vi "Check All.vi"(8 "error in (no error)":errorcluster, 11 "Lamp Container in":refnum<class "Lamp Container.lvclass">) -> (0 "error out":errorcluster, 3 "Lamp Container out":refnum<class "Lamp Container.lvclass">)   [LabVIEW 2016, in "Lamp Container.lvclass"]
uses:
  Lamp Container.lvclass
  Lamp Container.lvclass/Lamp Container.ctl
  ThAr/ThAr.lvclass
  LED/LED.lvclass
  Quartz/Quartz.lvclass
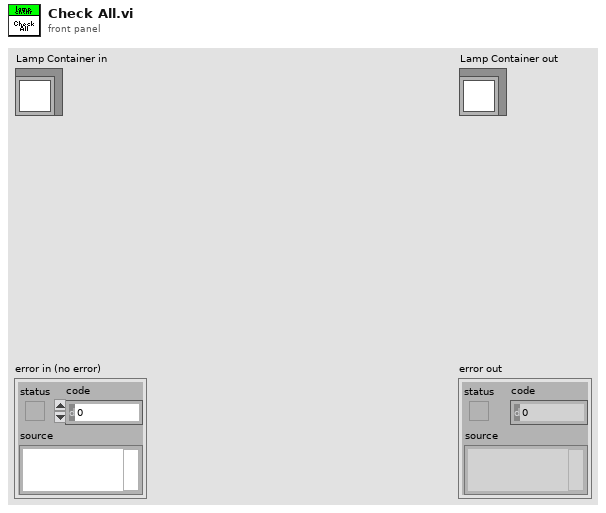
[diagram p1: front panel]
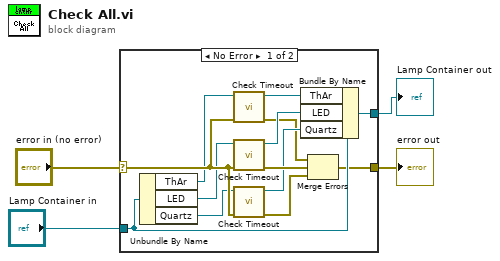
[diagram p0: block diagram]
diagram:
  n1 = case shown="No Error" "error in (no error)" {
    selector: "error in (no error)" -> [w14 w19]
    tunnel: [w15 w19] -> w3
    tunnel: [w16 w18] -> w1
    tunnel: "Lamp Container in" -> [w17 w18]
    frame No Error {
      n2 = Unbundle By Name(w17) -> ("ThAr"=w12:refnum<class "ThAr.lvclass">, "LED"=w13:refnum<class "LED.lvclass">, "Quartz"=w11:refnum<class "Quartz.lvclass">)
      n3 = call-dynamic "Check Timeout.vi"("error in (no error)"=w14, "Lamp in"=w12) -> ("error out"=w5:errorcluster, "Lamp out"=w6:refnum<class "ThAr.lvclass">)  [unwired: 8 in]
      n4 = call-dynamic "Check Timeout.vi"("error in (no error)"=w14, "Lamp in"=w13) -> ("error out"=w10:errorcluster, "Lamp out"=w7:refnum<class "LED.lvclass">)  [unwired: 8 in]
      n5 = call-dynamic "Check Timeout.vi"("error in (no error)"=w14, "Lamp in"=w11) -> ("error out"=w9:errorcluster, "Lamp out"=w8:refnum<class "Quartz.lvclass">)  [unwired: 8 in]
      n6 = Bundle By Name(cluster=w17, "ThAr"=w6, "LED"=w7, "Quartz"=w8) -> (w16:refnum<class "Lamp Container.lvclass">)
      n7 = Merge Errors(w5, w10, w9) -> (w15:errorcluster)
    }
    frame Error {
    }
  }
  "error out" <- w3
  "Lamp Container out" <- w1
